vi "onInterruptProcessTriggers.vi"(8 "error in (no error)":errorcluster, 10 "IAModel":refnum<class "IAModel.lvclass">, 11 "ConnectedState in":refnum<class "ConnectedState.lvclass">) -> (0 "error out":errorcluster, 2 "IAModel":refnum<class "IAModel.lvclass">, 3 "ConnectedState out":refnum<class "ConnectedState.lvclass">)   [LabVIEW 2016]
uses:
  _ComponentElements/ElementDomeSupervisor/ElementAClasses/IModel/IAModel.lvclass
  _ComponentElements/ElementDomeSupervisor/ElementAClasses/States/States/ConnectedState/ConnectedState.lvclass
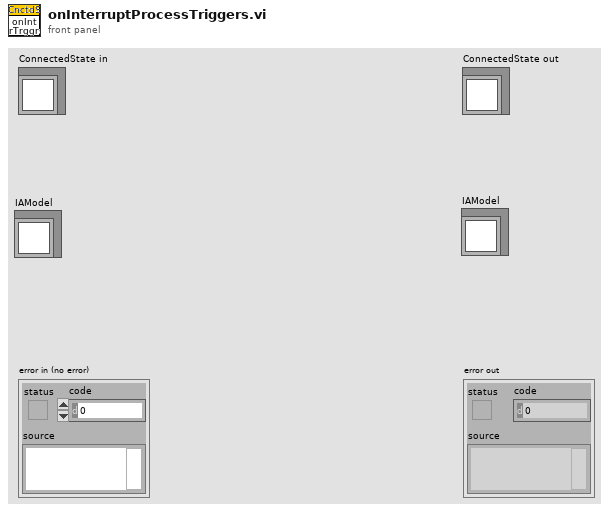
[diagram p1: front panel]
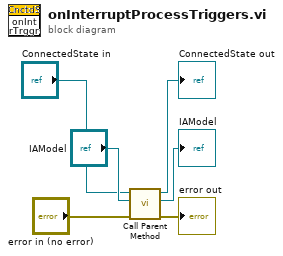
[diagram p0: block diagram]
diagram:
  n1 = call-parent "Call Parent Method"("error in (no error)"="error in (no error)", "IAModel"="IAModel", "AState in"="ConnectedState in") -> ("error out"=→"error out":errorcluster, "IAModel"=→"IAModel":refnum<class "IAModel.lvclass">, "AState out"=→"ConnectedState out":refnum<class "ConnectedState.lvclass">)  [unwired: 6 in]
